vi "ROI entry-ROI text overlay optimise.vi"(9 "ROI properties":T1 {"ROI group ID" format="%#_6f"; "Laser Power (%)" format="%#_6f"; "Zoom" format="%#_6f"; "Frame Size" format="%#_6f"; "Number of lines" format="%#_6f"; "Composite ID" format="%#_6f"; "Angle (deg)" format="%#_6f"; "ROI Time (ns)" format="%#_6f"; "ROI ID" format="%#_6f"; "Pixels in ROI" format="%#_6f"; "ROI index" format="%#_6f"; "Z stop" format="%#_6f"; "Y stop" format="%#_6f"; "X stop" format="%#_6f"; "Z start" format="%#_6f"; "X start" format="%#_6f"; "Y start" format="%#_6f"}, 11 "XY coordinates":cluster{"X":i32, "Y":i32}) -> (3 "XY coordinates":cluster{"X":i32, "Y":i32})   [LabVIEW 2017]
uses:
  Visualisation/Functional Imaging Viewer/Typedefs/ROI parameters data type.ctl
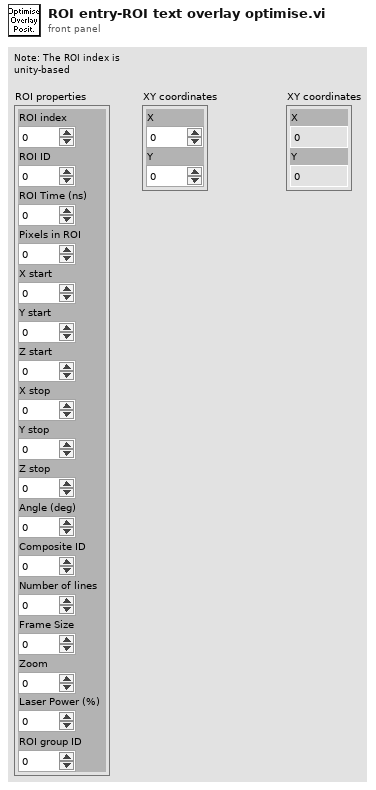
[diagram p1: front panel]
types:
  T1 = typedef "ROI parameters data type.ctl" = cluster{"ROI index":dbl, "ROI ID":dbl, "ROI Time (ns)":dbl, "Pixels in ROI":dbl, "X start":dbl, "Y start":dbl, "Z start":dbl, "X stop":dbl, "Y stop":dbl, "Z stop":dbl, "Angle (deg)":dbl, "Composite ID":dbl, "Number of lines":dbl, "Frame Size":dbl, "Zoom":dbl, "Laser Power (%)":dbl, "ROI group ID":dbl}
  T2 = typedef "ROI ID Enum.ctl" = enum16{"Point", "MiniScan", "Comp. MiniScan", "Rectangle", "Comp. volume", "Arb. plane point"}
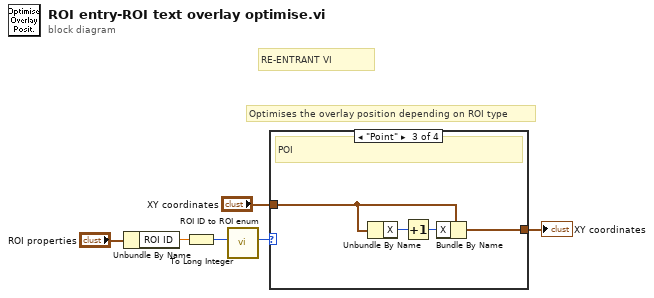
[diagram p0: block diagram]
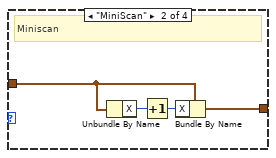
[diagram p3: hidden frame]
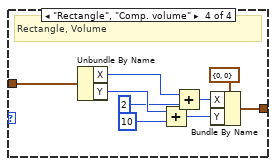
[diagram p4: hidden frame]
diagram:
  # "RE-ENTRANT VI"
  # "Optimises the overlay position depending on ROI type"
  n1 = Unbundle By Name("ROI properties") -> ("ROI ID"=w4:dbl)
  n2 = To Long Integer(number=w4) -> (32bit integer=w3:i32)
  n3 = call "ROI ID to ROI enum.vi"("ROI ID"=w3) -> ("ROI Enum"=w1:T2)  [unwired: 6 in]
  n4 = case shown="\"Point\"" w1 {
    tunnel: "XY coordinates" -> [w7 w9 w13 w22]
    tunnel: [w7 w8 w12 w17] -> w6
    frame Default {
    }
    frame "MiniScan" {
      # "Miniscan"
      n5 = Unbundle By Name(w9) -> ("X"=w10:i32)
      n6 = Increment(x=w10) -> (x+1=w11:i32)
      n7 = Bundle By Name(cluster=w9, "X"=w11) -> (w8:cluster{"X":i32, "Y":i32})
    }
    frame "Point" {
      # "POI"
      n8 = Unbundle By Name(w13) -> ("X"=w14:i32)
      n9 = Increment(x=w14) -> (x+1=w15:i32)
      n10 = Bundle By Name(cluster=w13, "X"=w15) -> (w12:cluster{"X":i32, "Y":i32})
    }
    frame "Rectangle", "Comp. volume" {
      # "Rectangle, Volume"
      n11 = Unbundle By Name(w22) -> ("X"=w23:i32, "Y"=w24:i32)
      n12 = Add(x=w24, y=10) -> (x+y=w19:i32)
      n13 = Add(x=w23, y=2) -> (x+y=w18:i32)
      n14 = Bundle By Name(cluster=cluster{"X":i32, "Y":i32} {"X"=0, "Y"=0} ("Point"), "X"=w18, "Y"=w19) -> (w17:cluster{"X":i32, "Y":i32})
    }
  }
  "XY coordinates" <- w6
